vi "Set Item Property Adapt For Scalar.vi"(6 "Set String as Binary":bool=TRUE, 8 "error in (no error)":errorcluster, 9 "Value":variant, 10 "Property Name":string, 11 "CDBase":refnum<k24>) -> (0 "error out":errorcluster, 2 "Replaced":bool, 3 "CDBase":refnum<k24>)   [LabVIEW 2020, in "Custom Device Offline API.lvlib"]
uses:
  <vilib>/NI VeriStand/Custom Device Offline API/Custom Device Offline API.lvlib
  NationalInstruments.VeriStand.SystemDefinitionAPI
  <vilib>/Utility/VariantDataType/VariantType.lvlib
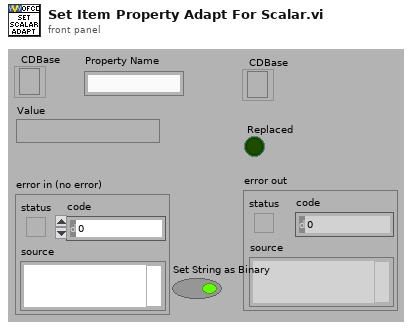
[diagram p1: front panel]
types:
  T1 = typedef "VariantType.lvlib/Type.ctl" = enum8{"Invalid Type", "Void", "I8", "I16", "I32", "I64", "U8", "U16", "U32", "U64", "Single Float", "Double Float", "Extended Float", "Single Complex", "Double Complex", "Extended Complex", "Enum U8", "Enum U16", "Enum U32", "Enum U64", "Single Float With Unit", "Double Float With Unit", "Extended Float With Unit", "Single Complex with Unit", "Double Complex with Unit", "Extended Complex with Unit", "Boolean", "String", "Path", "Picture", "Tag", "Array", "Cluster", "Variant", "LV Variant", "Waveform", "Timestamp", "Digital Waveform", "Digital Data", "ExpressData", "Refnum", "External Data", "VI", "Poly VI", "LabVIEW Class Instance", "Fixed Point"}
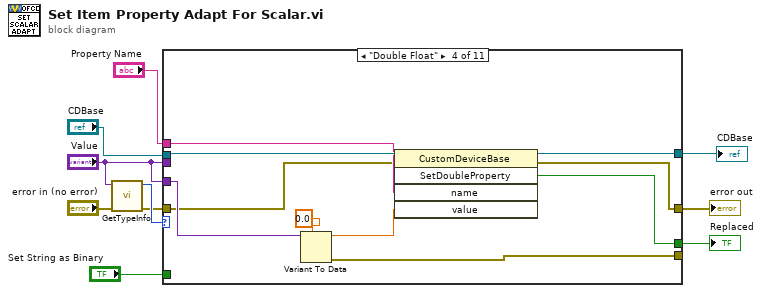
[diagram p0: block diagram]
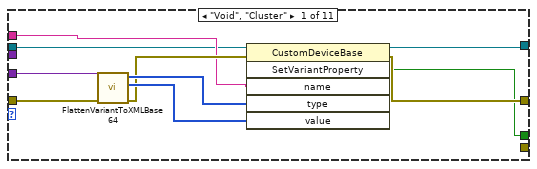
[diagram p2: hidden frame]
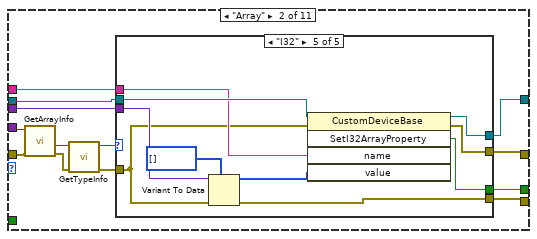
[diagram p3: hidden frame]
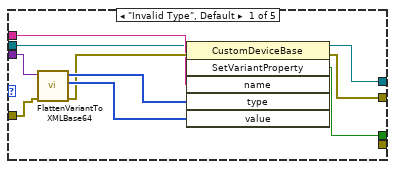
[diagram p4: hidden frame]
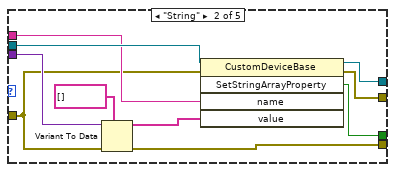
[diagram p5: hidden frame]
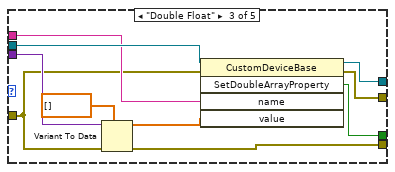
[diagram p6: hidden frame]
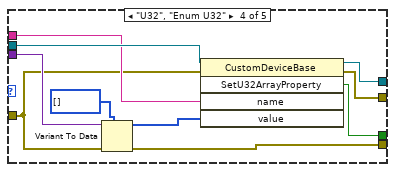
[diagram p7: hidden frame]
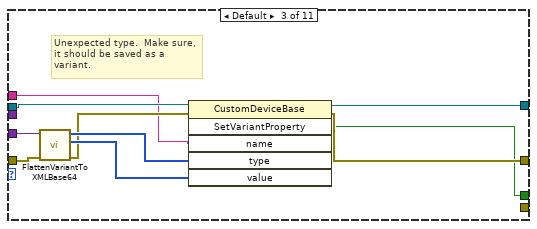
[diagram p8: hidden frame]
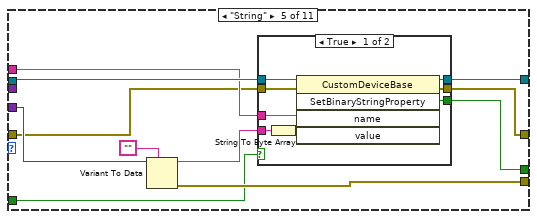
[diagram p9: hidden frame]
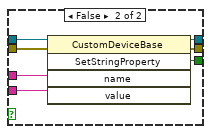
[diagram p10: hidden frame]
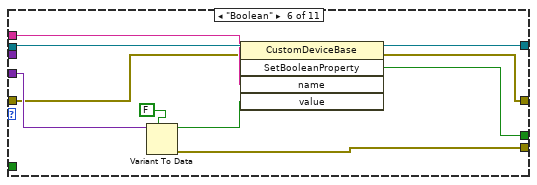
[diagram p11: hidden frame]
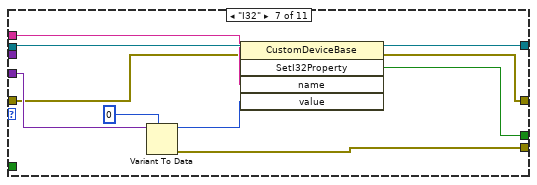
[diagram p12: hidden frame]
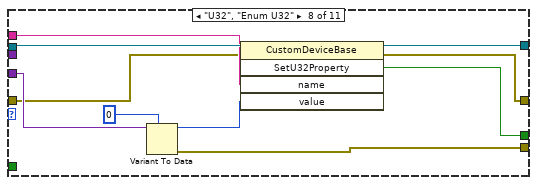
[diagram p13: hidden frame]
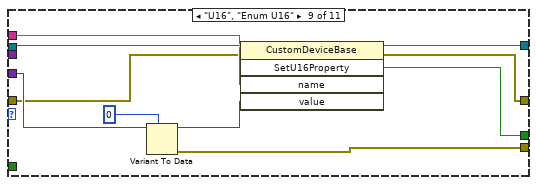
[diagram p14: hidden frame]
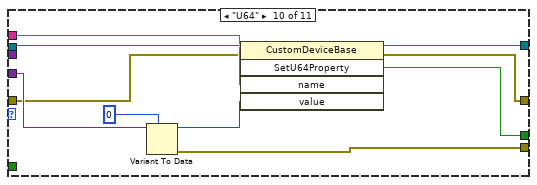
[diagram p15: hidden frame]
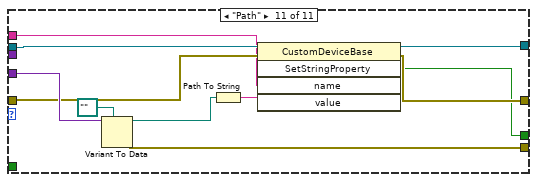
[diagram p16: hidden frame]
diagram:
  n1 = call <vilib>:"GetTypeInfo.vi"("error in (no error)"="error in (no error)", "Variant"="Value") -> ("error out"=w5:errorcluster, "Type Enum"=w10:T1)  [unwired: 5 in, 3 out]
  n2 = case shown="\"Double Float\"" w10 {
    tunnel: "CDBase" -> [w16 w26 w93 w100 w112 w136 w146 w156 w166 w176 w187]
    tunnel: w5 -> [w15 w32 w89 w98 w110 w134 w144 w154 w164 w174 w186]
    tunnel: [w13 w24 w86 w97 w109 w133 w143 w153 w163 w173 w182] -> w8
    tunnel: "Property Name" -> [w17 w25 w87 w99 w111 w135 w145 w155 w165 w175 w184]
    tunnel: "Value" -> [w14 w33 w92 w103 w114 w139 w149 w159 w169 w179 w190]
    tunnel: [w12 w23 w85 w96 w108 w132 w142 w152 w162 w172 w181] -> w7
    tunnel: [_ w22 _ w101 w113 w137 w147 w157 w167 w177 w185] -> _
    tunnel: "Value" -> [_ w27 _ _ _ _ _ _ _ _ _]
    tunnel: [w11 w21 w84 w94 w106 w130 w140 w150 w160 w170 w180] -> w2
    tunnel: "Set String as Binary" -> [_ _ _ _ w104 _ _ _ _ _ _]
    frame "Void", "Cluster" {
      n3 = call <vilib>:"FlattenVariantToXMLBase64.vi"("error in (no error)"=w15, "Variant"=w14) -> ("error out"=w18:errorcluster, "data"=w19:u8[], "type string"=w20:u8[])  [unwired: 7 in]
      n4 = invoke class="CustomDeviceBase" method="SetVariantProperty"(reference=w16, error in=w18, "name"=w17, "type"=w20, "value"=w19) -> (reference out=w11:refnum<k24>, error out=w13:errorcluster, "SetVariantProperty"=w12:bool)  [unwired: 1 in, 3 out]
    }
    frame "Array" {
      n5 = call <vilib>:"GetArrayInfo.vi"("error in (no error)"=w32, "Variant"=w33) -> ("error out"=w30:errorcluster, "ArrayElement"=w31:variant)  [unwired: 6 in, 2 out]
      n6 = call <vilib>:"GetTypeInfo.vi"("error in (no error)"=w30, "Variant"=w31) -> ("error out"=w28:errorcluster, "Type Enum"=w29:T1)  [unwired: 5 in, 3 out]
      n7 = case shown="\"I32\"" w29 {
        tunnel: w28 -> [w37 w46 w58 w67 w78]
        tunnel: w27 -> [w38 w53 w63 w73 w83]
        tunnel: w26 -> [w39 w50 w61 w71 w81]
        tunnel: w25 -> [w40 w48 w59 w69 w79]
        tunnel: [w36 w49 w60 w70 w80] -> w21
        tunnel: [w35 w44 w56 w65 w76] -> w24
        tunnel: [w34 w45 w57 w66 w77] -> w23
        tunnel: [_ w51 w62 w72 w82] -> w22
        frame "Invalid Type", Default {
          n8 = call <vilib>:"FlattenVariantToXMLBase64.vi"("error in (no error)"=w37, "Variant"=w38) -> ("error out"=w41:errorcluster, "data"=w42:u8[], "type string"=w43:u8[])  [unwired: 7 in]
          n9 = invoke class="CustomDeviceBase" method="SetVariantProperty"(reference=w39, error in=w41, "name"=w40, "type"=w43, "value"=w42) -> (reference out=w36:refnum<k24>, error out=w35:errorcluster, "SetVariantProperty"=w34:bool)  [unwired: 1 in, 3 out]
        }
        frame "String" {
          n10 = Variant To Data(error in=w46, type=string[] [], Variant=w53) -> (data=w47:string[], error out=w51:errorcluster)
          n11 = invoke class="CustomDeviceBase" method="SetStringArrayProperty"(reference=w50, error in=w46, "name"=w48, "value"=w47) -> (reference out=w49:refnum<k24>, error out=w44:errorcluster, "SetStringArrayProperty"=w45:bool)  [unwired: 1 in, 2 out]
        }
        frame "Double Float" {
          n12 = Variant To Data(error in=w58, type=dbl[] [], Variant=w63) -> (data=w54:dbl[], error out=w62:errorcluster)
          n13 = invoke class="CustomDeviceBase" method="SetDoubleArrayProperty"(reference=w61, error in=w58, "name"=w59, "value"=w54) -> (reference out=w60:refnum<k24>, error out=w56:errorcluster, "SetDoubleArrayProperty"=w57:bool)  [unwired: 1 in, 2 out]
        }
        frame "U32", "Enum U32" {
          n14 = Variant To Data(error in=w67, type=u32[] [], Variant=w73) -> (data=w68:u32[], error out=w72:errorcluster)
          n15 = invoke class="CustomDeviceBase" method="SetU32ArrayProperty"(reference=w71, error in=w67, "name"=w69, "value"=w68) -> (reference out=w70:refnum<k24>, error out=w65:errorcluster, "SetU32ArrayProperty"=w66:bool)  [unwired: 1 in, 2 out]
        }
        frame "I32" {
          n16 = Variant To Data(error in=w78, type=i32[] [], Variant=w83) -> (data=w74:i32[], error out=w82:errorcluster)
          n17 = invoke class="CustomDeviceBase" method="SetI32ArrayProperty"(reference=w81, error in=w78, "name"=w79, "value"=w74) -> (reference out=w80:refnum<k24>, error out=w76:errorcluster, "SetI32ArrayProperty"=w77:bool)  [unwired: 1 in, 2 out]
        }
      }
    }
    frame Default {
      # "Unexpected type.  Make sure, it should be saved as a variant."
      n18 = call <vilib>:"FlattenVariantToXMLBase64.vi"("error in (no error)"=w89, "Variant"=w92) -> ("error out"=w88:errorcluster, "data"=w90:u8[], "type string"=w91:u8[])  [unwired: 7 in]
      n19 = invoke class="CustomDeviceBase" method="SetVariantProperty"(reference=w93, error in=w88, "name"=w87, "type"=w91, "value"=w90) -> (reference out=w84:refnum<k24>, error out=w86:errorcluster, "SetVariantProperty"=w85:bool)  [unwired: 1 in, 3 out]
    }
    frame "Double Float" {
      n20 = Variant To Data(type=0.0, Variant=w103) -> (data=w95:dbl, error out=w101:errorcluster)  [unwired: 1 in]
      n21 = invoke class="CustomDeviceBase" method="SetDoubleProperty"(reference=w100, error in=w98, "name"=w99, "value"=w95) -> (reference out=w94:refnum<k24>, error out=w97:errorcluster, "SetDoubleProperty"=w96:bool)  [unwired: 1 in, 2 out]
    }
    frame "String" {
      n22 = Variant To Data(type="", Variant=w114) -> (data=w107:string, error out=w113:errorcluster)  [unwired: 1 in]
      n23 = case shown="True" w104 {
        tunnel: w112 -> [w122 w129]
        tunnel: w111 -> [w121 w128]
        tunnel: w110 -> [w120 w127]
        tunnel: [w119 w126] -> w109
        tunnel: [w118 w125] -> w108
        tunnel: w107 -> [w117 w124]
        tunnel: [w116 w123] -> w106
        frame True {
          n24 = String To Byte Array(string=w117) -> (unsigned byte array=w115:u8[])
          n25 = invoke class="CustomDeviceBase" method="SetBinaryStringProperty"(reference=w122, error in=w120, "name"=w121, "value"=w115) -> (reference out=w116:refnum<k24>, error out=w119:errorcluster, "SetBinaryStringProperty"=w118:bool)  [unwired: 1 in, 2 out]
        }
        frame False {
          n26 = invoke class="CustomDeviceBase" method="SetStringProperty"(reference=w129, error in=w127, "name"=w128, "value"=w124) -> (reference out=w123:refnum<k24>, error out=w126:errorcluster, "SetStringProperty"=w125:bool)  [unwired: 1 in, 2 out]
        }
      }
    }
    frame "Boolean" {
      n27 = Variant To Data(type=FALSE, Variant=w139) -> (data=w131:bool, error out=w137:errorcluster)  [unwired: 1 in]
      n28 = invoke class="CustomDeviceBase" method="SetBooleanProperty"(reference=w136, error in=w134, "name"=w135, "value"=w131) -> (reference out=w130:refnum<k24>, error out=w133:errorcluster, "SetBooleanProperty"=w132:bool)  [unwired: 1 in, 2 out]
    }
    frame "I32" {
      n29 = Variant To Data(type=0, Variant=w149) -> (data=w141:i32, error out=w147:errorcluster)  [unwired: 1 in]
      n30 = invoke class="CustomDeviceBase" method="SetI32Property"(reference=w146, error in=w144, "name"=w145, "value"=w141) -> (reference out=w140:refnum<k24>, error out=w143:errorcluster, "SetI32Property"=w142:bool)  [unwired: 1 in, 2 out]
    }
    frame "U32", "Enum U32" {
      n31 = Variant To Data(type=u32 0, Variant=w159) -> (data=w151:u32, error out=w157:errorcluster)  [unwired: 1 in]
      n32 = invoke class="CustomDeviceBase" method="SetU32Property"(reference=w156, error in=w154, "name"=w155, "value"=w151) -> (reference out=w150:refnum<k24>, error out=w153:errorcluster, "SetU32Property"=w152:bool)  [unwired: 1 in, 2 out]
    }
    frame "U16", "Enum U16" {
      n33 = Variant To Data(type=u16 0, Variant=w169) -> (data=w161:u16, error out=w167:errorcluster)  [unwired: 1 in]
      n34 = invoke class="CustomDeviceBase" method="SetU16Property"(reference=w166, error in=w164, "name"=w165, "value"=w161) -> (reference out=w160:refnum<k24>, error out=w163:errorcluster, "SetU16Property"=w162:bool)  [unwired: 1 in, 2 out]
    }
    frame "U64" {
      n35 = Variant To Data(type=u64 0, Variant=w179) -> (data=w171:u64, error out=w177:errorcluster)  [unwired: 1 in]
      n36 = invoke class="CustomDeviceBase" method="SetU64Property"(reference=w176, error in=w174, "name"=w175, "value"=w171) -> (reference out=w170:refnum<k24>, error out=w173:errorcluster, "SetU64Property"=w172:bool)  [unwired: 1 in, 2 out]
    }
    frame "Path" {
      n37 = Variant To Data(type=path "", Variant=w190) -> (data=w188:path, error out=w185:errorcluster)  [unwired: 1 in]
      n38 = Path To String(path=w188) -> (string=w183:string)
      n39 = invoke class="CustomDeviceBase" method="SetStringProperty"(reference=w187, error in=w186, "name"=w184, "value"=w183) -> (reference out=w180:refnum<k24>, error out=w182:errorcluster, "SetStringProperty"=w181:bool)  [unwired: 1 in, 2 out]
    }
  }
  "Replaced" <- w7
  "error out" <- w8
  "CDBase" <- w2
